vi "05 - Dataset Lifecycle.vi"() -> ()   [LabVIEW 2020]
uses:
  client/client.lvlib
panel:
  out "dataset created found":bool
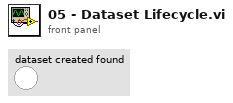
[diagram p1: front panel]
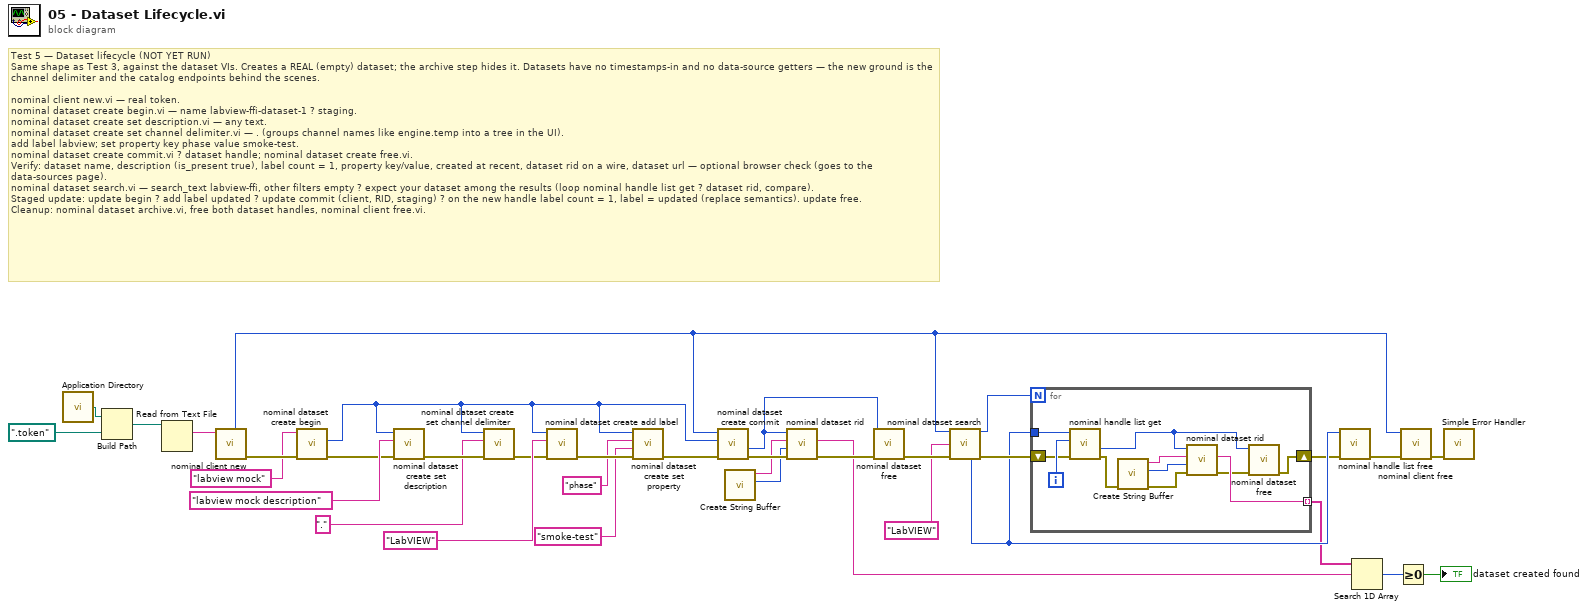
[diagram p0: block diagram]
diagram:
  # "Test 5 — Dataset lifecycle (NOT YET RUN)\nSame shape as Test 3, against the dataset VIs. Creates a REAL (empty) dataset; the archive step hides it. Datasets have no timestamps-in and no data-source getters — the new ground is the channel delimiter and the catalog endpoints behind the scenes.\n\nnominal client new.vi — real token.\nnominal dataset create begin.vi — name labview-ffi-dataset-1 ? staging.\nnominal dataset create set description.vi — any text.\nnominal dataset create set channel delimiter.vi — . (groups channel names like engine.temp into a tree in the UI).\nadd label labview; set property key phase value smoke-test.\nnominal dataset create commit.vi ? dataset handle; nominal dataset create free.vi.\nVerify: dataset name, description (is_present true), label count = 1, property key/value, created at recent, dataset rid on a wire, dataset url — optional browser check (goes to the data-sources page).\nnominal dataset search.vi — search_text labview-ffi, other filters empty ? expect your dataset among the results (loop nominal handle list get ? dataset rid, compare).\nStaged update: update begin ? add label updated ? update commit (client, RID, staging) ? on the new handle label count = 1, label = updated (replace semantics). update free.\nCleanup: nominal dataset archive.vi, free both dataset handles, nominal client free.vi."
  n1 = call <vilib>:"Application Directory.vi"() -> ("Application Directory"=w34:path)
  n2 = Build Path(base path=w34, name or relative path=path ".token") -> (appended path=w32:path)
  n3 = Read from Text File(file (use dialog)=w32) -> (text=w31:string)  [unwired: 3 in, 3 out]
  n4 = call "nominal client new.vi"("token"=w31) -> ("error out"=w30:errorcluster, "out_client out"=w17:i32)  [unwired: 8 in, 1 out]
  n5 = call "nominal dataset create begin.vi"("error in (no error)"=w30, "name"="labview mock") -> ("error out"=w27:errorcluster, "out_staging out"=w19:i32)  [unwired: 7 in, 1 out]
  n6 = call "nominal dataset create set description.vi"("error in (no error)"=w27, "description"="labview mock description" ("name"), "staging"=w19) -> ("error out"=w26:errorcluster)  [unwired: 7 in, 1 out]
  n7 = call "nominal dataset create set channel delimiter.vi"("error in (no error)"=w26, "delimiter"="." ("name"), "staging"=w19) -> ("error out"=w23:errorcluster)  [unwired: 7 in, 1 out]
  n8 = call "nominal dataset create add label.vi"("error in (no error)"=w23, "label"="LabVIEW" ("name"), "staging"=w19) -> ("error out"=w22:errorcluster)  [unwired: 7 in, 1 out]
  n9 = call "nominal dataset create set property.vi"("error in (no error)"=w22, "value"="smoke-test" ("name"), "key"="phase" ("name"), "staging"=w19) -> ("error out"=w18:errorcluster)  [unwired: 6 in, 1 out]
  n10 = call "nominal dataset create commit.vi"("error in (no error)"=w18, "staging"=w19, "client"=w17) -> ("error out"=w9:errorcluster, "out_dataset out"=w8:i32)  [unwired: 6 in, 1 out]
  n11 = call "Create String Buffer.vi"() -> ("dub Buffer Size"=w6:i32, "String Buffer"=w7:string)  [unwired: 9 in, 1 out]
  n12 = call "nominal dataset rid.vi"("error in (no error)"=w9, "cap"=w6, "buf"=w7, "dataset"=w8) -> ("error out"=w5:errorcluster, "buf out"=w3:string)  [unwired: 4 in, 2 out]
  n13 = call "nominal dataset free.vi"("error in (no error)"=w5, "dataset"=w8) -> ("error out"=w16:errorcluster)  [unwired: 8 in, 1 out]
  n14 = call "nominal dataset search.vi"("client"=w17, "label"="LabVIEW", "error in (no error)"=w16) -> ("out_count out"=w14:u32, "out_list out"=w12:i32, "error out"=w13:errorcluster)  [unwired: 9 in, 1 out]
  n15 = for {
    N: w14 -> [_]
    tunnel: w12 -> [w46]
    shift-right: [w37] -> w11
    shift-left: w13 -> [w44]
    tunnel: [w39] -> w4 mode=indexing
    i -> [w45]
    n16 = call "nominal handle list get.vi"("error in (no error)"=w44, "index"=w45, "list"=w46) -> ("error out"=w43:errorcluster, "out_handle out"=w36:i32)  [unwired: 6 in, 1 out]
    n17 = call "Create String Buffer.vi"("error in"=w43) -> ("error out"=w42:errorcluster, "dub Buffer Size"=w41:i32, "String Buffer"=w40:string)  [unwired: 8 in]
    n18 = call "nominal dataset rid.vi"("error in (no error)"=w42, "cap"=w41, "buf"=w40, "dataset"=w36) -> ("error out"=w38:errorcluster, "buf out"=w39:string)  [unwired: 4 in, 2 out]
    n19 = call "nominal dataset free.vi"("error in (no error)"=w38, "dataset"=w36) -> ("error out"=w37:errorcluster)  [unwired: 8 in, 1 out]
  }
  n20 = call "nominal handle list free.vi"("error in (no error)"=w11, "list"=w12) -> ("error out"=w10:errorcluster)  [unwired: 8 in, 1 out]
  n21 = Search 1D Array(1D array=w4, element=w3) -> (index of element=w2:i32)  [unwired: 1 in]
  n22 = Greater Or Equal To 0?(x=w2) -> (x >= 0?=→"dataset created found":bool)
  n23 = call "nominal client free.vi"("error in (no error)"=w10, "client"=w17) -> ("error out"=w35:errorcluster)  [unwired: 8 in, 1 out]
  n24 = call <vilib>:"Simple Error Handler.vi"("error in (no error)"=w35) -> ()  [unwired: 4 in, 5 out]
